vi "Wire Selected_Index To Case Selector.vi"(8 "error in (no error)":errorcluster, 9 "CaseStructure in":refnum<vi>, 10 "SubVI in":refnum<vi>, 11 "Unbundler in":refnum<vi>) -> (0 "error out":errorcluster, 1 "Case Structure out":refnum<vi>, 2 "SubVI out":refnum<vi>, 3 "Unbundler out":refnum<vi>)   [LabVIEW 2019, in "gRPC Template Creation Utility.lvlib"]
uses:
  gRPC Template Creation Utility.lvlib
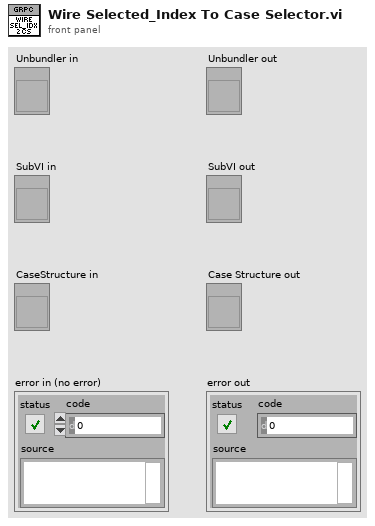
[diagram p1: front panel]
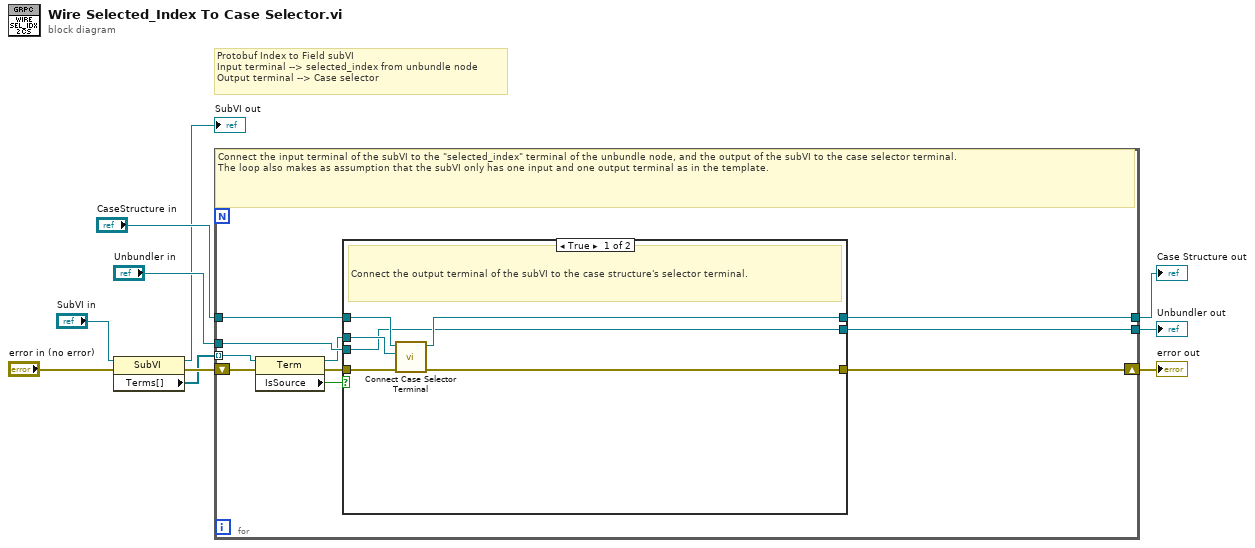
[diagram p0: block diagram]
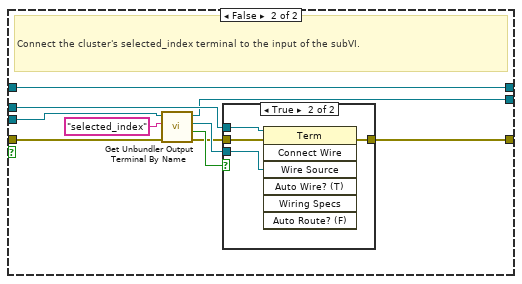
[diagram p2: hidden frame]
diagram:
  # "Protobuf Index to Field subVI\nInput terminal --> selected_index from unbundle node\nOutput terminal --> Case selector"
  n1 = property class="SubVI"(reference="SubVI in", error in="error in (no error)") -> (reference out=→"SubVI out":refnum<vi>, error out=w10:errorcluster, "Terms[]"=w6:refnum<vi>[])
  n2 = for {
    tunnel: w6 -> [w16] mode=indexing
    tunnel: "Unbundler in" -> [w19]
    tunnel: "CaseStructure in" -> [w15]
    shift-right: [w14] -> w9
    shift-left: w10 -> [w13]
    tunnel: [w12] -> w2
    tunnel: [w11] -> w1
    # "Connect the input terminal of the subVI to the \"selected_index\" terminal of the unbundle node, and the output of the subVI to the case selector terminal.\nThe loop also makes as assumption that the subVI only has one input and one output terminal as in the template."
    n3 = property class="Term"(reference=w16, error in=w13) -> (reference out=w17:refnum<vi>, error out=w18:errorcluster, "IsSource"=w20:bool)
    n4 = case shown="True" w20 {
      tunnel: w19 -> [w21 w36]
      tunnel: w18 -> [w24 w35]
      tunnel: w17 -> [w25 w34]
      tunnel: w15 -> [w26 w28]
      tunnel: [w23 w30] -> w14
      tunnel: [w22 w28] -> w12
      tunnel: [w21 w27] -> w11
      frame True {
        # "Connect the output terminal of the subVI to the case structure's selector terminal."
        n5 = call "Connect Case Selector Terminal.vi"("error in (no error)"=w24, "Wire Source"=w25, "Case Structure in"=w26) -> ("error IO"=w23:errorcluster, "Case Structure out"=w22:refnum<vi>)  [unwired: 7 in]
      }
      frame False {
        # "Connect the cluster's selected_index terminal to the input of the subVI."
        n6 = call "Get Unbundler Output Terminal By Name.vi"("error in (no error)"=w35, "Terminal name"="selected_index" ("String"), "Unbundler in"=w36) -> ("error out"=w31:errorcluster, "Found?"=w32:bool, "Terminal Refnum"=w33:refnum<vi>, "Unbundler out"=w27:refnum<vi>)  [unwired: 5 in]
        n7 = case shown="True" w32 {
          tunnel: w34 -> [_ w41]
          tunnel: w33 -> [_ w40]
          tunnel: w31 -> [w37 w39]
          tunnel: [w37 w38] -> w30
          frame False {
          }
          frame True {
            n8 = invoke class="Term" method="Connect Wire"(reference=w41, error in=w39, "Wire Source"=w40) -> (error out=w38:errorcluster)  [unwired: 4 in, 6 out]
          }
        }
      }
    }
  }
  "error out" <- w9
  "Case Structure out" <- w2
  "Unbundler out" <- w1
